vi "Play Pause.vi"(8 "error in (no error)":errorcluster, 10 "Play Pause":bool, 11 "[V] Main UI in":refnum<class "[V] Main UI.lvclass">) -> (0 "error out":errorcluster, 3 "[V] Main UI out":refnum<class "[V] Main UI.lvclass">)   [LabVIEW 2020, in "[V] Main UI.lvlib" / "[V] Main UI.lvclass"]
uses:
  [V] Main UI.lvclass
  C:/Program Files (x86)/National Instruments/LabVIEW 2020/vi.lib/ActorFramework/Actor/Actor.lvclass
  [V] Main UI.lvclass/[V] Main UI.ctl
  <vilib>/ActorFramework/Actor/Actor.lvclass/Actor.ctl
  <vilib>/ActorFramework/Message Enqueuer/Message Enqueuer.lvclass/Message Enqueuer.ctl
  [V] Main UI Messages/Play Pause Msg/Play Pause Msg.lvclass/Play Pause Msg.ctl
  Controls/Play Pause.ctl
  <vilib>/ActorFramework/Message Enqueuer/Init from Existing Queue.vi
  <vilib>/ActorFramework/Message Enqueuer/Enqueue.vi
  [V] Main UI Messages/Play Pause Msg/Play Pause Msg.lvclass
  C:/Program Files (x86)/National Instruments/LabVIEW 2020/vi.lib/ActorFramework/Message/Message.lvclass
  <vilib>/ActorFramework/Message Priority Queue/Priority Enqueue.vi
  <vilib>/ActorFramework/Message Enqueuer/Message Enqueuer.lvclass
  <vilib>/ActorFramework/Actor/Actor.lvclass
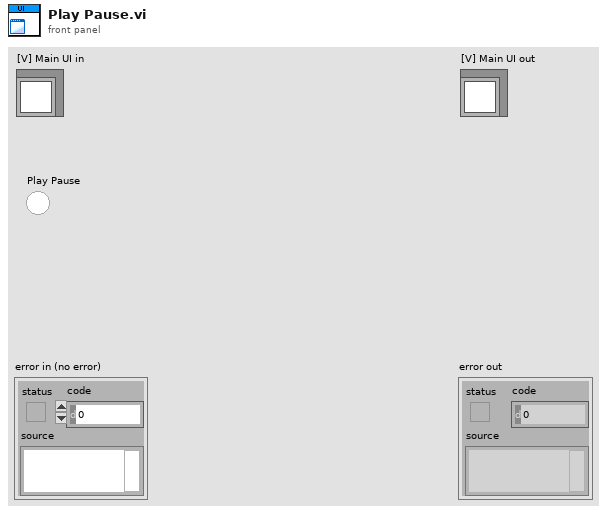
[diagram p1: front panel]
types:
  T1 = typedef "Play Pause.ctl" = bool
  T2 = typedef "number.ctl" = i8
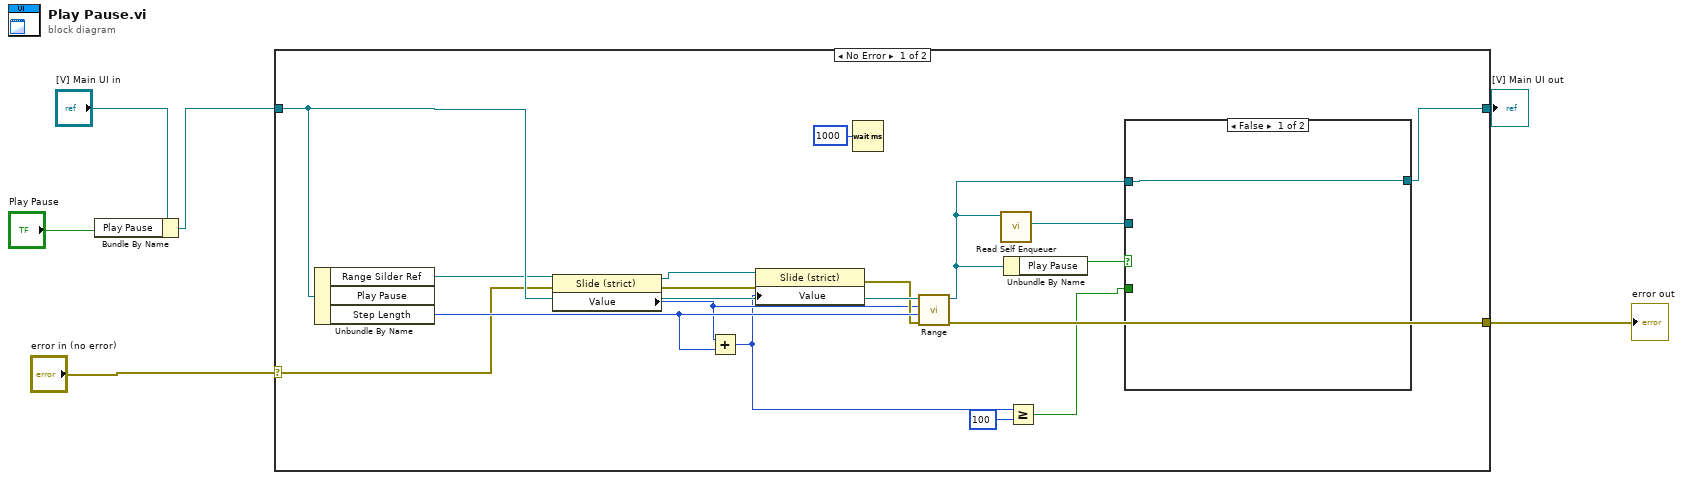
[diagram p0: block diagram]
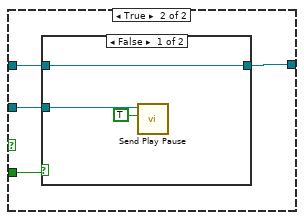
[diagram p2: hidden frame]
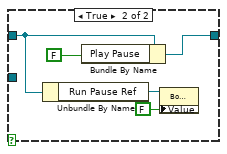
[diagram p3: hidden frame]
diagram:
  n1 = Bundle By Name(cluster="[V] Main UI in", "Play Pause"="Play Pause") -> (w1:refnum<class "[V] Main UI.lvclass">)
  n2 = case shown="No Error" "error in (no error)" {
    selector: "error in (no error)" -> [w20 w38]
    tunnel: [w19 w38] -> w5
    tunnel: [w7 w37] -> w4
    tunnel: w1 -> [w23 w37]
    frame No Error {
      n3 = Unbundle By Name(w23) -> ("Range Silder Ref"=w22:refnum<vi>, "Step Length"=w21:u8)  [unwired: 1 out]
      n4 = property class="Slide (strict)"(reference=w22, error in=w20) -> (reference out=w16:refnum<vi>, error out=w15:errorcluster, "Value"=w13:T2)
      n5 = Add(x=w13, y=w21) -> (x+y=w11:u8)
      n6 = property class="Slide (strict)"(reference=w16, error in=w15, "Value"=w11) -> (error out=w14:errorcluster)  [unwired: 1 out]
      n7 = Wait (ms)(milliseconds to wait=u32 1000) -> ()  [unwired: 1 out]
      n8 = call "Range.vi"("error in (no error)"=w14, "length"=w21, "index"=w13, "[V] Main UI in"=w23) -> ("error out"=w19:errorcluster, "[V] Main UI out"=w8:refnum<class "[V] Main UI.lvclass">)  [unwired: 6 in]
      n9 = call <vilib>:"Read Self Enqueuer.vi"("Actor"=w8) -> ("Self Enqueuer"=w12:refnum<class "Message Enqueuer.lvclass">)  [unwired: 10 in]
      n10 = Unbundle By Name(w8) -> ("Play Pause"=w18:bool)
      n11 = Greater Or Equal?(x=w11, y=u8 100) -> (x >= y?=w9:bool)
      n12 = case shown="False" w18 {
        tunnel: w12 -> [_ w28]
        tunnel: w9 -> [_ w27]
        tunnel: w8 -> [w24 w26]
        tunnel: [w24 w25] -> w7
        frame False {
        }
        frame True {
          n13 = case shown="False" w27 {
            tunnel: w28 -> [w31 _]
            tunnel: w26 -> [w30 w34]
            tunnel: [w30 w35] -> w25
            frame False {
              n14 = call "Send Play Pause.vi"("Play Pause"=TRUE, "Message Enqueuer"=w31) -> ()  [unwired: 8 in, 2 out]
            }
            frame True {
              n15 = Unbundle By Name(w34) -> ("Run Pause Ref"=w33:refnum<vi>)
              n16 = Bundle By Name(cluster=w34, "Play Pause"=FALSE) -> (w35:refnum<class "[V] Main UI.lvclass">)
              n17 = property class="Bool (strict)"(reference=w33, "Value"=T1 FALSE) -> ()  [unwired: 1 in, 2 out]
            }
          }
        }
      }
    }
    frame Error {
    }
  }
  "error out" <- w5
  "[V] Main UI out" <- w4
